vi "Global Tree Data.vi"() -> ()   [LabVIEW 2020, in "Sequencer with Output Values.lvlib" / "Sequencer with Output Values.lvclass"]
uses:
  Sequencer with Output Values.lvclass
  Tree Item Settings.ctl
  Data Type.ctl
panel:
  in  "Description - Step":string="This is a step in the sequence. Use the settings under this item to configure how long the step will last and any values to assign to channels while the step is active."
  in  "Description - Digital Values":string="These are the values the channel will have during the step. Use a semi-colon to specify more than one value. For digital lines, only 0 and 1 are supported. Use the \"Delay Between Values (s)\" to determine how long to wait between values. Use the \"Mode to determine what to do if these values complete before the end of the step."
  in  "Description - Analog Values":string="These are the values the channel will have during the step. Use a semi-colon to specify more than one value. Use the \"Delay Between Values (s)\" to determine how long to wait between values. Use the \"Mode to determine what to do if these values complete before the end of the step."
  in  "Description - Delay Between Values":string="This determines how much delay to wait between values on the channels. If 0 is specified, the values will automatically be interpolated over the duration of the step. This value applies to all the analog and digital channels within the step. Each step can have a different delay and values for the channels."
  in  "Digital Chan Val Index":i32=11
  in  "Mode Index":i32=8
  in  "Analog Chan Val Index":i32=10
  in  "Step Index":i32=6
  in  "Description - Mode":string="This determines how to handle channel values that complete before the duration of the step. \"Wait for end of step\" will keep the last channel value until the step ends. \"Repeat channel values\" will start at the beginning of the channel values and continue repeating until the step ends."
  in  "Description - Duration":string="This determines how long the sequence will remain in this step until changing to the next step. If any channel values are defined that would last longer than this duration, they will be cut short since this step will always last exactly this duration. "
  in  "Description - Reset Sequence When Test Starts":string="This determines if the sequence should reset when the test starts. This option has no effect when \"Only Execute When Test is Running\" is true since the sequence will always reset when the test starts regardless of this option."
  in  "Description - Only Execute When Test Running":string="This determines if the sequence should execute only when the test is running. When this is true, the sequence will not start executing until the test begins and the sequence will also pause and resume when the test pauses and resumes. When this is false, the sequence is always executing. The \"Time Left\" channel will not have valid data until the sequence begins, but it will keep it's last value while the test is paused."
  in  "Description - Delay After Test Start":string="This determines how much time in seconds to wait before executing the sequence after a test starts. It only applies if \"Only execute when test is running\" is true or \"Reset sequence when test starts\" is true. When there is a delay, the \"Time Left\" channel will not have valid data until the sequence begins."
  in  "Description - Number of Digital Channels":string="The number of digital channels to define for each step of the sequence. These channels can be mapped to DAQmx or other boolean output channels to control their value as the sequence changes."
  in  "Description - Number of Analog Channels":string="The number of analog channels to define for each step of the sequence. These channels can be mapped to DAQmx or other numeric output channels to control their value as the sequence changes."
  in  "Description - Number of Steps":string="The number of sequence steps. Each step can have a duration and set values for analog or digital lines. The sequence will repeat after the last step is complete."
  in  "False":string="False"
  in  "True":string="True"
  in  "Tree Label Constants":T1[](array[typedef])=[{"Indent Level"=0, "Data Type"=0, "Numeric Range"={"Min"=1.0, "Max"=100.0, "Inc"=1.0}, "Enum Values"=[], "Default Value"="1"}, {"Indent Level"=0, "Data Type"=0, "Numeric Range"={"Min"=0.0, "Max"=10.0, "Inc"=1.0}, "Enum Values"=[], "Default Value"="0"}, {"Indent Level"=0, "Data Type"=0, "Numeric Range"={"Min"=0.0, "Max"=10.0, "Inc"=1.0}, "Enum Values"=[], "Default Value"="0"}, {"Indent Level"=0, "Data Type"=0, "Numeric Range"={"Min"=0.0, "Max"=1000.0, "Inc"=0.0}, "Enum Values"=[], "Default Value"="0"}, {"Indent Level"=0, "Data Type"=2, "Numeric Range"={"Min"=0.0, "Max"=0.0, "Inc"=0.0}, "Enum Values"=[], "Default Value"="False"}, {"Indent Level"=0, "Data Type"=2, "Numeric Range"={"Min"=0.0, "Max"=0.0, "Inc"=0.0}, "Enum Values"=[], "Default Value"="True"}, {"Indent Level"=0, "Data Type"=-1, "Numeric Range"={"Min"=0.0, "Max"=0.0, "Inc"=0.0}, "Enum Values"=[], "Default Value"="0"}, {"Indent Level"=1, "Data Type"=0, "Numeric Range"={"Min"=0.1, "Max"=100000.0, "Inc"=0.1}, "Enum Values"=[], "Default Value"="1"}, {"Indent Level"=1, "Data Type"=3, "Numeric Range"={"Min"=0.0, "Max"=0.0, "Inc"=0.0}, "Enum Values"=["Wait for end of step", "Repeat channel values"], "Default Value"="Wait for end of step"}, {"Indent Level"=1, "Data Type"=0, "Numeric Range"={"Min"=0.0, "Max"=100000.0, "Inc"=0.1}, "Enum Values"=[], "Default Value"=".1"}, {"Indent Level"=1, "Data Type"=1, "Numeric Range"={"Min"=0.0, "Max"=0.0, "Inc"=0.0}, "Enum Values"=[], "Default Value"="0"}, {"Indent Level"=1, "Data Type"=1, "Numeric Range"={"Min"=0.0, "Max"=0.0, "Inc"=0.0}, "Enum Values"=[], "Default Value"="0"}] {"Data Type" items=["Tree Parent"=-1, "Numeric"=0, "String"=1, "Boolean"=2, "Enum"=3]}
  in  "Tree Labels":string[](array[string])=["Number of sequence steps", "Number of analog channels", "Number of digital channels", "Delay after test starts (sec)", "Only execute when test is running", "Reset sequence when test starts", "Step %d", "Duration (sec)", "Mode", "Delay between values (sec)", "Analog channel %d values", "Digital channel %d values"]
  # "These are fixed"
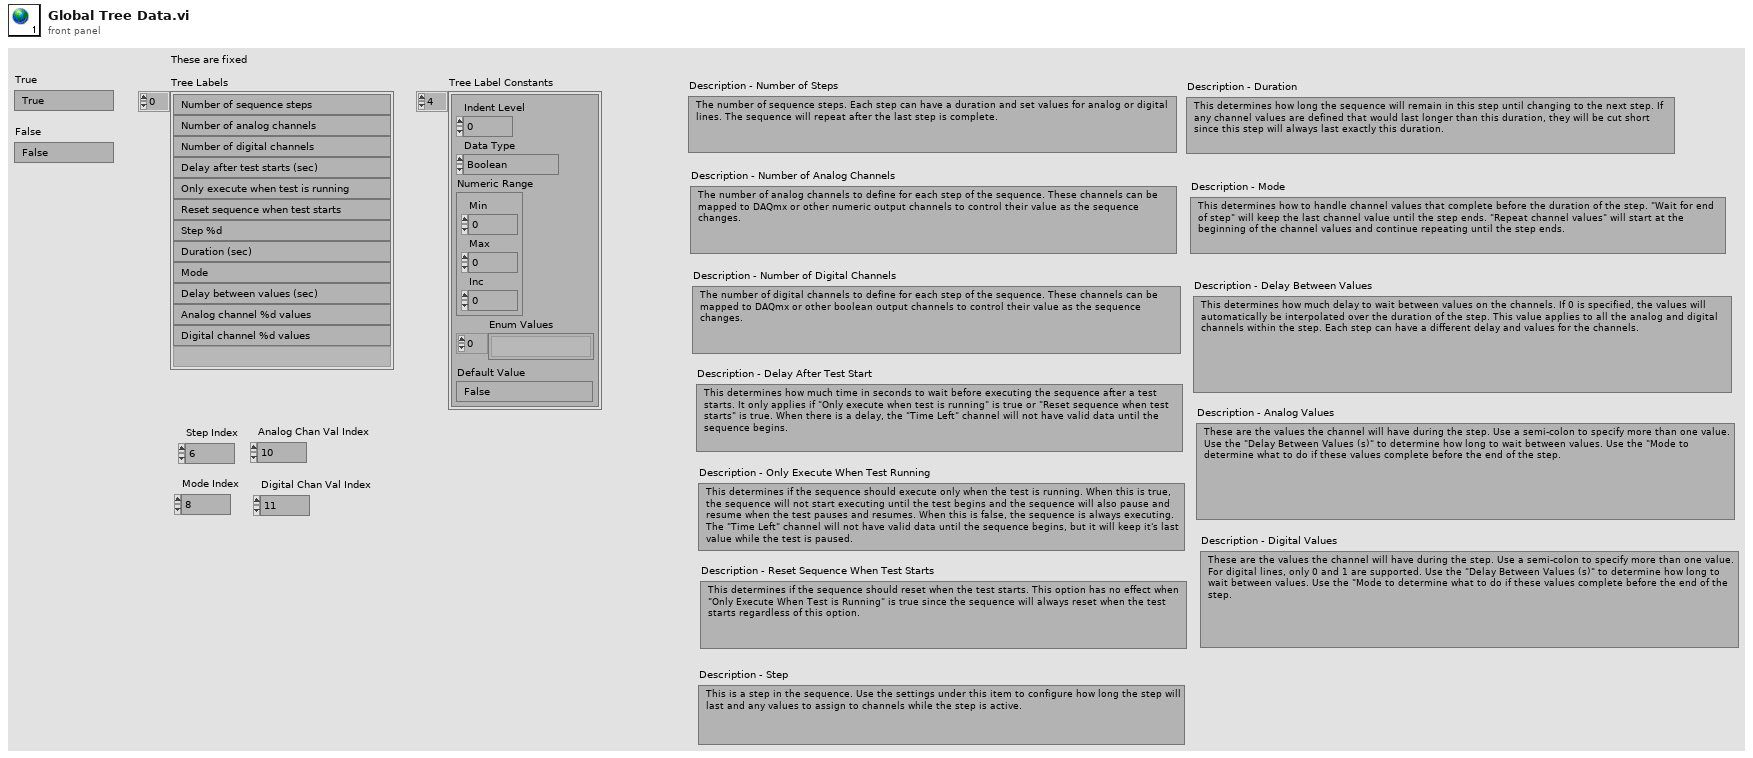
[diagram p1: front panel]
types:
  T1 = typedef "Sequencer with Output Values.lvlib/Sequencer with Output Values.lvclass/Tree Item Settings.ctl" = cluster{"Indent Level":i32, "Data Type":T2, "Numeric Range":cluster{"Min":dbl, "Max":dbl, "Inc":dbl}, "Enum Values":string[], "Default Value":string}
  T2 = typedef "Sequencer with Output Values.lvlib/Sequencer with Output Values.lvclass/Data Type.ctl" = i16
diagram:
